vi "TLB Native Dynamic Events ver 0.09a.vi"() -> ()   [LabVIEW 2018]
uses:
  Labview Training Phase 2/Enum Controls/States for Action Engine.ctl
  Type def/TLB event states.ctl
  Type def/TLB MHL States.ctl
  <vilib>/Studica/Studica Toolkit/Background/I2C Channel.ctl
  <vilib>/myRIO/Common/Instrument Driver Framework/myRIO v1.0/AI/typedefs/AI Channels Enum.ctl
  <vilib>/myRIO/Common/Instrument Driver Framework/myRIO v1.0/AI/typedefs/AI Channels List.ctl
  Type def/Type def.ctl
  Underlying VI's/Webcam FGV Low level ver/State control.ctl
  <vilib>/userdefined/High Color/IMAQdx.ctl
  <vilib>/Studica/Studica Toolkit/NavX/NavX.lvlib
  <vilib>/Studica/Studica Toolkit/Background/DIO Channel.ctl
panel:
  out "State Queue Items":T1[](array[typedef])
  in  "NavX LED":bool
  out "Speed & distance":T2
  out "Motor Error":errorcluster
  in  "Direction":T3(ring)
  in  "Speed":dbl(slide) scale=-120.0..120.0
  out "I2C Error":errorcluster
  out "NavX Error":errorcluster
  out "Raw Values":T4
  out "NavX Data":T5
  out "Arduino Data":T6
  in  "STOP TASK":bool
  in  "Select task":i8
  in  "OK Button":bool
  out "Yaw":dbl
  out "Decision":i8
  in  "STOP":bool
  out "error out":errorcluster
  out "Object detection count":T7
  out "Camera error":errorcluster
  out "element":T1
  out "Action Queue Items":i32
  out "State Logic Queue Items":i32
  out "Action Queues items":string[](array[string])=["Hardware reset", "Software reset", ""]
  out "State logic":T8=enum."Task 2"
  out "Action State":string
  # "TLB FRAMEWORK STATUS"
  # "Camera Status Loop"
  # "Test Programme written by Calvin Loke    Dated: 28 Aug 2019\nTest Programme revised by Dr Alex See   Dated 30 Aug 2019\n\nProgramme version:   TLB Native Dynamic Events ver 0.04b.vi"
  # "Motor Control Loop"
  # "NAVX Control Loop"
  # "System Health Status Update"
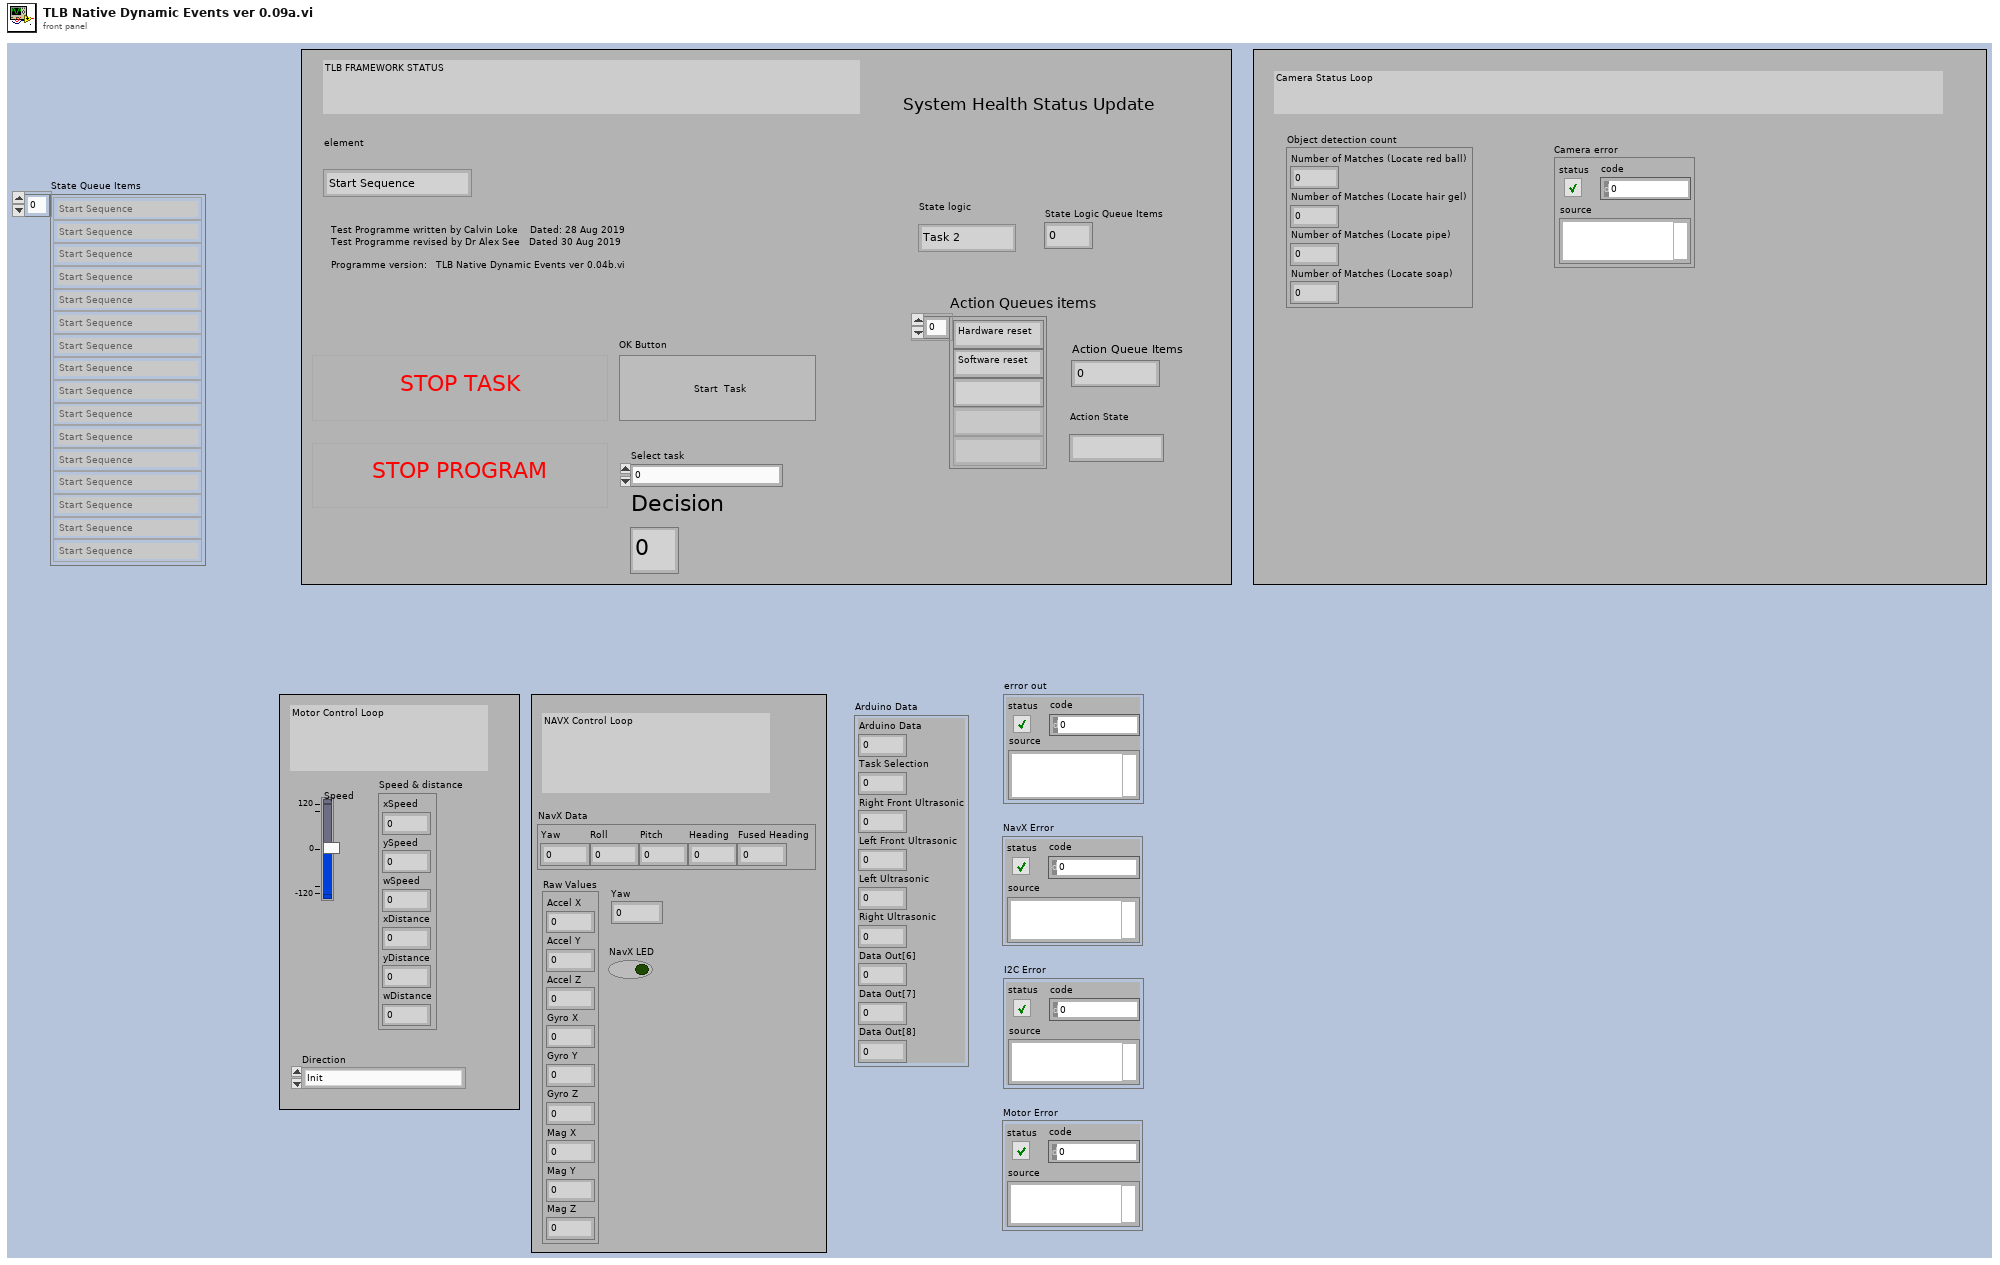
[diagram p1: front panel]
types:
  T1 = typedef "TLB event states.ctl" = enum16{"Start Sequence", "Exit", "Start Task 1", "Start Task 2", "Start Task 3", "Start Task 4", "Camera vision", "Wall follow mode", "Idle", "Start Drive Straight"}
  T2 = cluster{"xSpeed":dbl, "ySpeed":dbl, "wSpeed":dbl, "xDistance":dbl, "yDistance":dbl, "wDistance":dbl}
  T3 = enum16{"Init", "Front Back", "Left Right", "Rotate", "Latch"}
  T4 = cluster{"Accel X":dbl, "Accel Y":dbl, "Accel Z":dbl, "Gyro X":dbl, "Gyro Y":dbl, "Gyro Z":dbl, "Mag X":dbl, "Mag Y":dbl, "Mag Z":dbl}
  T5 = cluster{"Yaw":dbl, "Roll":dbl, "Pitch":dbl, "Heading":dbl, "Fused Heading":dbl}
  T6 = cluster{"Arduino Data":u8, "Task Selection":u8, "Right Front Ultrasonic":u8, "Left Front Ultrasonic":u8, "Left Ultrasonic":u8, "Right Ultrasonic":u8, "Data Out[6]":u8, "Data Out[7]":u8, "Data Out[8]":u8}
  T7 = cluster{"Number of Matches (Locate red ball)":i32, "Number of Matches (Locate hair gel)":i32, "Number of Matches (Locate pipe)":i32, "Number of Matches (Locate soap)":i32}
  T8 = typedef "TLB MHL States.ctl" = enum16{"None", "Startup", "Idle", "Processing", "Shutdown", "Reset", "Task 1", "Task 2", "Task 3", "Task 4", "Task 4a", "Task 4b", "Task 4c", "Task 4d", "Task 4e", "Task 4f", "Task 4g", "Task 4h", "Acquire image", "Wall follow mode", "Autodrive", "Autodrive a"}
  T9 = typedef "States for Action Engine.ctl" = enum16{"Initialize", "Write", "Read"}
  T10 = typedef "DIO Channel.ctl" = enum16{"Not Connected", "A/DIO1", "A/DIO2", "A/DIO3", "A/DIO4", "A/DIO5", "A/DIO6", "A/DIO7", "A/DIO13", "B/DIO1", "B/DIO2", "B/DIO3", "B/DIO4", "B/DIO5", "B/DIO6", "B/DIO7", "B/DIO13", "C/DIO0", "C/DIO1", "C/DIO2", "C/DIO3", "C/DIO4", "C/DIO5", "C/DIO6", "C/DIO7"}
  T11 = typedef "Type def.ctl" = cluster{"Front Ultrasonic Obstruct":bool, "Left Ultrasonic Obstruct":bool, "Right Ultrasonic Obstruct ":bool}
  T12 = typedef "I2C Channel.ctl" = enum16{"Not Connected", "A", "B"}
  T13 = typedef "State control.ctl" = enum16{"Initialise", "Start camera", "Continuous Acquisition ", "Stop camera", "Dispose all"}
  T14 = typedef "IMAQdx.ctl" = refnum<k21>
  T15 = cluster{"DIO Channel":T10, "FPGA VI Reference Out":refnum<k20>}
  T16 = typedef "AI Channels List.ctl" = T17[]
  T17 = typedef "AI Channels Enum.ctl" = enum16{"Not Connected", "AudioIn/Left", "AudioIn/Right", "C/AI0", "C/AI1", "A/AI0", "A/AI1", "A/AI2", "A/AI3", "A/AI4", "A/AI5", "A/AI6", "A/AI7", "B/AI0", "B/AI1", "B/AI2", "B/AI3", "B/AI4", "B/AI5", "B/AI6", "B/AI7", "AI/AI0", "AI/AI1", "AI/AI2", "AI/AI3", "A/AI0 (DIFF)", "A/AI1 (DIFF)", "A/AI2 (DIFF)", "A/AI3 (DIFF)", "B/AI0 (DIFF)", "B/AI1 (DIFF)", "B/AI2 (DIFF)", "B/AI3 (DIFF)"}
  T18 = cluster{"Arduino Status":u8, "Task Selection":u8, "PING_A":u8, "PING_B":u8, "PING_C":u8, "PING_D":u8, "Compass Low Byte":u8, "Compass High Byte":u8, "Data Out[8]":u8}
  T19 = cluster{"I2C Ref Out":cluster{"I2C Channel":T12, "FPGA VI Reference Out":refnum<k20>}, "Connected":bool, "Slave Address (7-bit)":u8, "Registry":u8[]}
  T20 = typedef "IMAQ Image.ctl" = refnum<image>
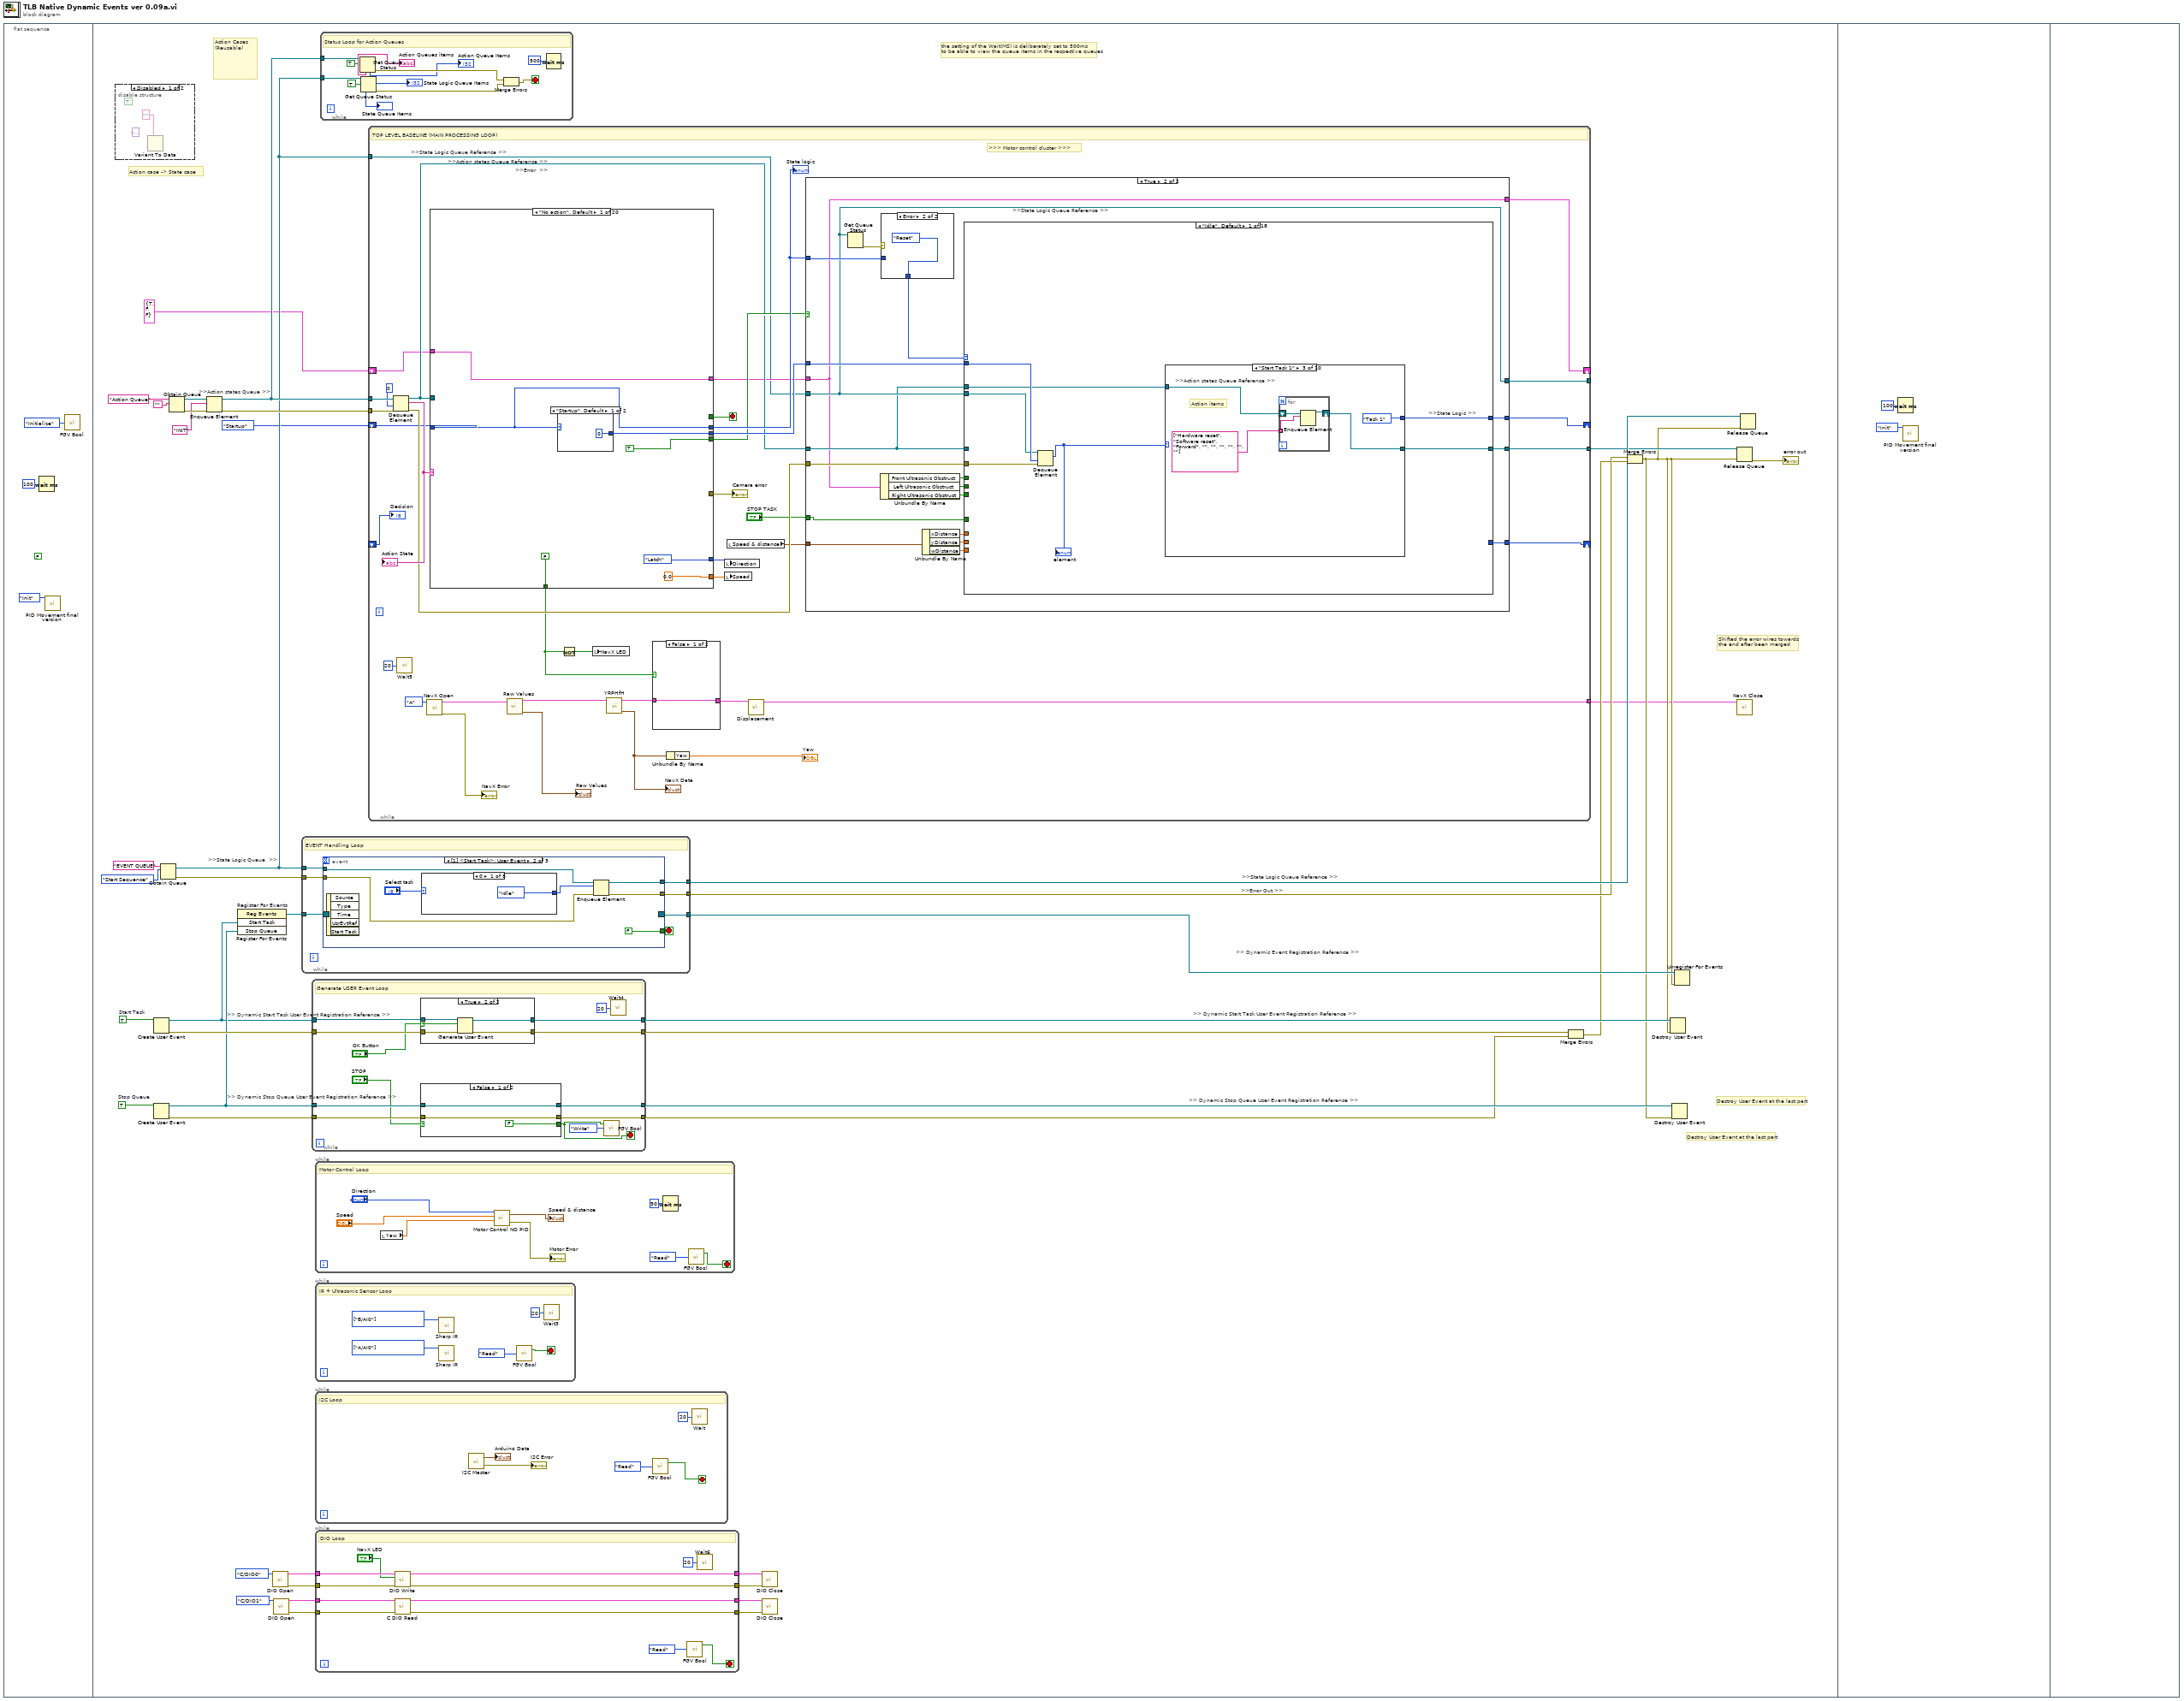
[diagram p0: block diagram]
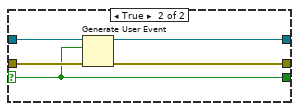
[diagram p3: hidden frame]
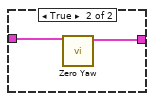
[diagram p5: hidden frame]
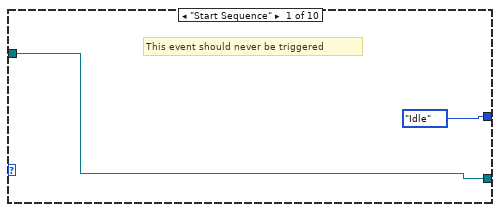
[diagram p8: hidden frame]
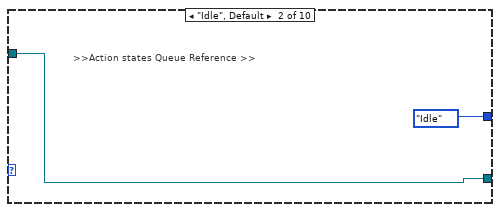
[diagram p9: hidden frame]
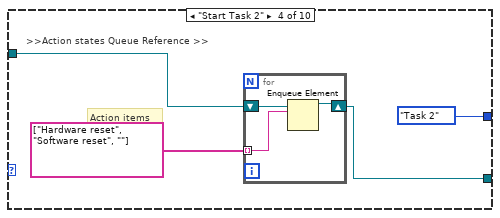
[diagram p10: hidden frame]
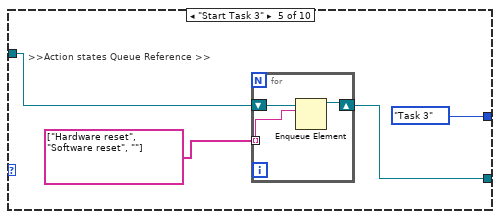
[diagram p11: hidden frame]
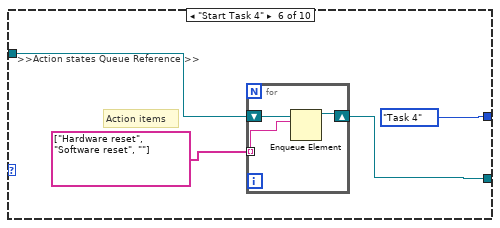
[diagram p12: hidden frame]
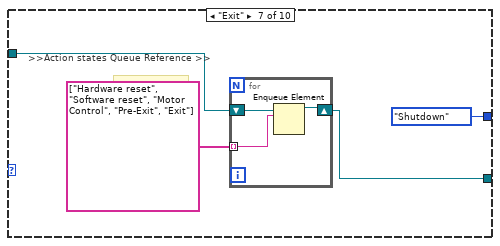
[diagram p13: hidden frame]
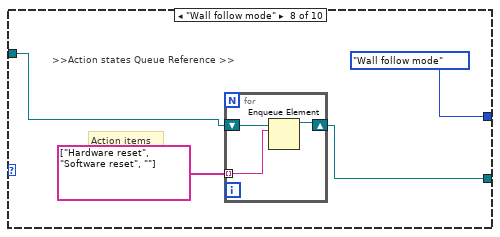
[diagram p14: hidden frame]
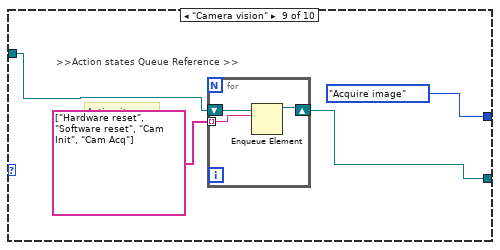
[diagram p15: hidden frame]
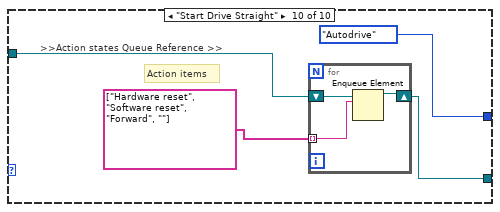
[diagram p16: hidden frame]
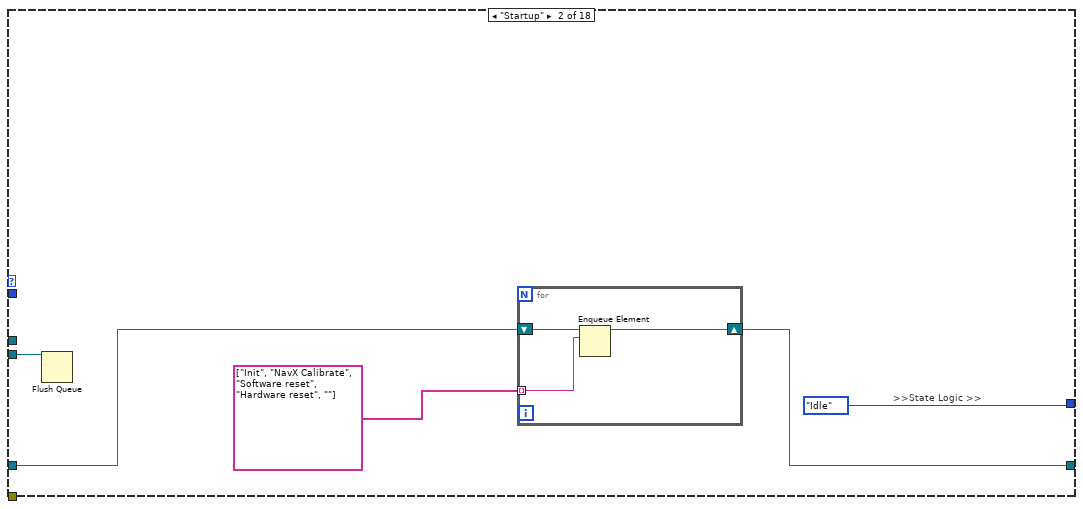
[diagram p17: hidden frame]
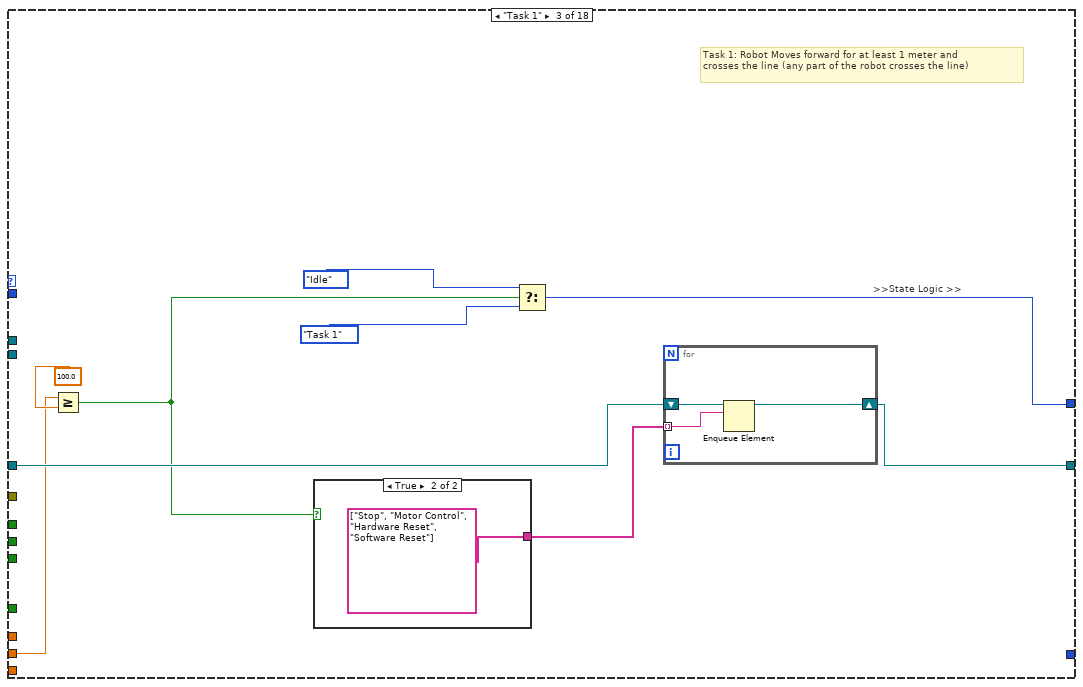
[diagram p18: hidden frame]
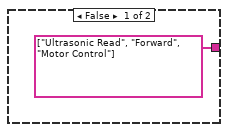
[diagram p19: hidden frame]
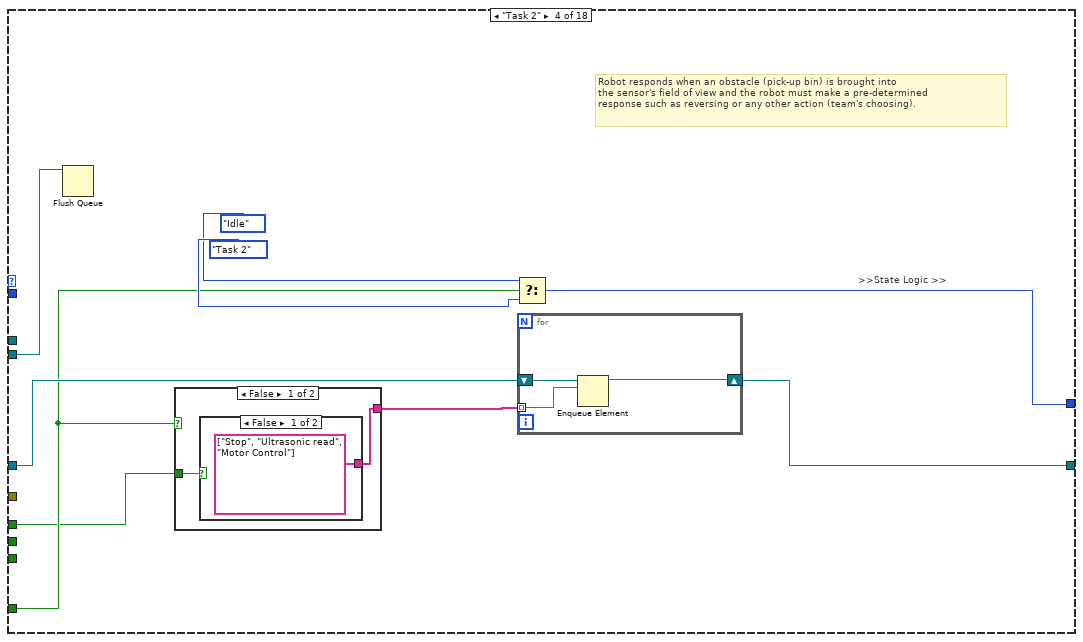
[diagram p20: hidden frame]
diagram:
  n1 = flat-sequence {
    frame #0 {
      (unwired) FALSE ("DIO 1")
      n2 = Wait (ms)(milliseconds to wait=u32 100) -> ()  [unwired: 1 out]
      n3 = call "PID Movement final version.vi"("Direction"=T3."Init") -> ()  [unwired: 3 in, 2 out]
      n4 = call "FGV Bool.vi"("Init/Read/Write State"=States_for_Action_Engine."Initialize") -> ()  [unwired: 2 in, 2 out]
    }
    frame #1 {
      w45 = TRUE  # Stop Queue
      w44 = TRUE  # Start Task
      # "Action case -> State case"
      # "the setting of the Wait(MS) is deliberately set to 500ms\nto be able to view the queue items in the respective queues"
      # "Action Cases\n(Reusable)"
      # ">>Error Out >>"
      # ">> Dynamic Stop Queue User Event Registration Reference >>"
      # ">> Dynamic Start Task User Event Registration Reference >>"
      # ">> Dynamic Stop Queue User Event Registration Reference >>"
      # ">> Dynamic Start Task User Event Registration Reference >>"
      # ">> Dynamic Event Registration Reference >>"
      # ">>Action states Queue >>"
      # ">>State Logic Queue  >>"
      # ">>State Logic Queue Reference >>"
      # "Destroy User Event at the last part"
      # "Destroy User Event at the last part"
      # "Shifted the error wires towards\nthe end after been merged"
      n5 = disable-structure shown="Disabled" {
        frame Disabled {
          (unwired) variant
          (unwired) TRUE
          n6 = Variant To Data(type="") -> ()  [unwired: 2 in, 2 out]
        }
        frame Enabled {
        }
      }
      n7 = Create User Event(user event datatype=w44) -> (user event=w36:refnum<user-event>, error out=w41:errorcluster)  [unwired: 1 in]
      n8 = Create User Event(user event datatype=w45) -> (user event=w37:refnum<user-event>, error out=w40:errorcluster)  [unwired: 1 in]
      n9 = Obtain Queue(name (unnamed)="EVENT QUEUE", element data type=TLB_event_states."Start Sequence" ("Enum")) -> (queue out=w21:refnum<queue>, error out=w27:errorcluster)  [unwired: 3 in, 1 out]
      n10 = Obtain Queue(name (unnamed)="Action Queue", element data type="") -> (queue out=w30:refnum<queue>, error out=w26:errorcluster)  [unwired: 3 in, 1 out]
      n11 = Enqueue Element(queue=w30, element="INIT", error in (no error)=w26) -> (queue out=w22:refnum<queue>, error out=w25:errorcluster)  [unwired: 1 in, 1 out]
      n12 = register-events "Register For Events"(w36, w37) -> (reference out=w35:refnum<event-registration>)  [unwired: 2 in, 1 out]
      n13 = call <vilib>:"DIO Open.vi"("DIO Channel"=DIO_Channel."C/DIO0") -> ("error out"=w11:errorcluster, "DIO Info Out"=w13:T15)  [unwired: 9 in]
      n14 = call <vilib>:"DIO Open.vi"("DIO Channel"=DIO_Channel."C/DIO1") -> ("error out"=w7:errorcluster, "DIO Info Out"=w8:T15)  [unwired: 9 in]
      n15 = while {
        tunnel: w35 -> [w637]
        tunnel: [w636] -> w34
        tunnel: w21 -> [w634]
        tunnel: [w633] -> w33
        tunnel: w27 -> [w632]
        tunnel: [w631] -> w24
        stop <- w635 stop-if-true
        # "EVENT Handling Loop"
        n16 = event shown="[1] <Start Task>: User Event" {
          selector: w637 -> [_ _ _]
          dyn-events: [_ _ _] -> w636
          timeout: _ -> [_ _ _]
          tunnel: [FALSE FALSE w664] -> w635
          tunnel: w634 -> [w642 w649 w662]
          tunnel: [w641 w648 w663] -> w633
          tunnel: w632 -> [w639 w647 w660]
          tunnel: [w638 w646 w659] -> w631
          event Timeout {
            n17 = event-data() -> ()  [unwired: 1 in, 3 out]
            n18 = Enqueue Element(queue=w642, element=TLB_event_states."Idle" ("Enum"), error in (no error)=w639) -> (queue out=w641:refnum<queue>, error out=w638:errorcluster)  [unwired: 1 in, 1 out]
          }
          event User Event {
            n19 = event-data() -> ()  [unwired: 1 in, 5 out]
            n20 = case shown="0" "Select task" {
              tunnel: [TLB_event_states."Idle" ("Enum") TLB_event_states."Start Task 1" ("Enum") TLB_event_states."Start Task 2" ("Enum") TLB_event_states."Start Task 3" ("Enum") TLB_event_states."Start Task 4" ("Enum") TLB_event_states."Wall follow mode" ("Enum") TLB_event_states."Camera vision" ("Enum") TLB_event_states."Start Drive Straight" ("Enum")] -> w645
              frame 0 {
              }
              frame 1 {
              }
              frame 2 {
              }
              frame 3, Default {
              }
              frame 4 {
              }
              frame 5 {
              }
              frame 6 {
              }
              frame 7 {
              }
            }
            n21 = Enqueue Element(queue=w649, element=w645, error in (no error)=w647) -> (queue out=w648:refnum<queue>, error out=w646:errorcluster)  [unwired: 1 in, 1 out]
          }
          event User Event {
            n22 = event-data() -> ("Stop Queue"=w664:bool)  [unwired: 1 in, 4 out]
            n23 = Enqueue Element At Opposite End(queue=w662, element=TLB_event_states."Exit" ("Enum"), error in (no error)=w660) -> (queue out=w663:refnum<queue>, error out=w659:errorcluster)  [unwired: 1 in, 1 out]
          }
        }
      }
      n24 = while {
        tunnel: w36 -> [w96]
        tunnel: w37 -> [w95]
        tunnel: [w94] -> w43
        tunnel: [w93] -> w42
        tunnel: w41 -> [w92]
        tunnel: [w91] -> w39
        tunnel: w40 -> [w90]
        tunnel: [w89] -> w38
        stop <- w87 stop-if-true
        # "Generate USER Event Loop"
        n25 = case shown="True" "OK Button" {
          selector: "OK Button" -> [_ w107]
          tunnel: w96 -> [w106 w111]
          tunnel: [w106 w110] -> w93
          tunnel: w92 -> [w105 w109]
          tunnel: [w105 w108] -> w91
          frame False {
          }
          frame True {
            n26 = Generate User Event(user event=w111, event data cluster=w107, error in=w109) -> (user event out=w110:refnum<user-event>, error out=w108:errorcluster)  [unwired: 1 in]
          }
        }
        n27 = case shown="False" "STOP" {
          selector: "STOP" -> [_ w100]
          tunnel: w95 -> [w99 w104]
          tunnel: [w99 w103] -> w94
          tunnel: w90 -> [w98 w102]
          tunnel: [w98 w101] -> w89
          tunnel: [FALSE w100] -> w87
          frame False {
          }
          frame True {
            n28 = Generate User Event(user event=w104, event data cluster=w100, error in=w102) -> (user event out=w103:refnum<user-event>, error out=w101:errorcluster)  [unwired: 1 in]
          }
        }
        n29 = call "FGV Bool.vi"("Init/Read/Write State"=States_for_Action_Engine."Write", "Input Node"=w87) -> ()  [unwired: 1 in, 2 out]
        n30 = call "Wait4"("Count(uSec)"=u32 20) -> ()  [unwired: 1 out]
      }
      n31 = while {
        stop <- w64 stop-if-true
        # "Motor Control Loop"
        n32 = local read "Yaw"() -> (w60:dbl)
        n33 = call "Motor Control NO PID.vi"("Yaw"=w60, "Speed"="Speed", "Direction"="Direction") -> ("error out"=→"Motor Error":errorcluster, "Speed & distance"=→"Speed & distance":T2)  [unwired: 1 in]
        n34 = Wait (ms)(milliseconds to wait=u32 50) -> ()  [unwired: 1 out]
        n35 = call "FGV Bool.vi"("Init/Read/Write State"=States_for_Action_Engine."Read") -> ("Output node"=w64:bool)  [unwired: 2 in, 1 out]
      }
      n36 = while {
        stop <- w627 stop-if-true
        w629 = T16 [enum."A/AI0"] items=["Not Connected", "AudioIn/Left", "AudioIn/Right", "C/AI0", "C/AI1", "A/AI0", "A/AI1", "A/AI2", "A/AI3", "A/AI4", "A/AI5", "A/AI6", "A/AI7", "B/AI0", "B/AI1", "B/AI2", "B/AI3", "B/AI4", "B/AI5", "B/AI6", "B/AI7", "AI/AI0", "AI/AI1", "AI/AI2", "AI/AI3", "A/AI0 (DIFF)", "A/AI1 (DIFF)", "A/AI2 (DIFF)", "A/AI3 (DIFF)", "B/AI0 (DIFF)", "B/AI1 (DIFF)", "B/AI2 (DIFF)", "B/AI3 (DIFF)"] ("AI Channel")
        w630 = T16 [enum."B/AI0"] items=["Not Connected", "AudioIn/Left", "AudioIn/Right", "C/AI0", "C/AI1", "A/AI0", "A/AI1", "A/AI2", "A/AI3", "A/AI4", "A/AI5", "A/AI6", "A/AI7", "B/AI0", "B/AI1", "B/AI2", "B/AI3", "B/AI4", "B/AI5", "B/AI6", "B/AI7", "AI/AI0", "AI/AI1", "AI/AI2", "AI/AI3", "A/AI0 (DIFF)", "A/AI1 (DIFF)", "A/AI2 (DIFF)", "A/AI3 (DIFF)", "B/AI0 (DIFF)", "B/AI1 (DIFF)", "B/AI2 (DIFF)", "B/AI3 (DIFF)"] ("AI Channel")
        # "IR + Ultrasonic Sensor Loop"
        n37 = call <vilib>:"Sharp IR.vi"("AI Channel"=w630) -> ()  [unwired: 8 in, 3 out]
        n38 = call <vilib>:"Sharp IR.vi"("AI Channel"=w629) -> ()  [unwired: 8 in, 3 out]
        n39 = call "FGV Bool.vi"("Init/Read/Write State"=States_for_Action_Engine."Read") -> ("Output node"=w627:bool)  [unwired: 2 in, 1 out]
        n40 = call "Wait3"("Count(uSec)"=u32 20) -> ()  [unwired: 1 out]
      }
      n41 = while {
        stop <- w69 stop-if-true
        # "I2C Loop"
        n42 = call "I2C Master.vi"() -> ("I2C Error"=→"I2C Error":errorcluster, "Arduino Data"=→"Arduino Data":T18)  [unwired: 2 in]
        n43 = call "FGV Bool.vi"("Init/Read/Write State"=States_for_Action_Engine."Read") -> ("Output node"=w69:bool)  [unwired: 2 in, 1 out]
        n44 = call "Wait"("Count(uSec)"=u32 20) -> ()  [unwired: 1 out]
      }
      n45 = while {
        tunnel: w13 -> [w54]
        tunnel: [w53] -> w12
        tunnel: w11 -> [w52]
        tunnel: [w51] -> w10
        tunnel: [w50] -> w9
        tunnel: w8 -> [w49]
        tunnel: w7 -> [w48]
        tunnel: [w47] -> w6
        stop <- w56 stop-if-true
        # "DIO Loop"
        n46 = call <vilib>:"DIO Write.vi"("error in (no error)"=w52, "Input"="NavX LED", "DIO Info In"=w54) -> ("error out"=w51:errorcluster, "DIO Info Out"=w53:T15)  [unwired: 7 in]
        n47 = call <vilib>:"C DIO Read.vi"("error in (no error)"=w48, "DIO Info In in"=w49) -> ("error out"=w47:errorcluster, "DIO Info In out"=w50:T15)  [unwired: 7 in, 1 out]
        n48 = call "FGV Bool.vi"("Init/Read/Write State"=States_for_Action_Engine."Read") -> ("Output node"=w56:bool)  [unwired: 2 in, 1 out]
        n49 = call "Wait6"("Count(uSec)"=u32 20) -> ()  [unwired: 1 out]
      }
      n50 = while {
        tunnel: w22 -> [w81]
        tunnel: w21 -> [w78]
        stop <- w75 stop-if-true
        # "Status Loop for Action Queues"
        n51 = Get Queue Status(queue=w81, return elements? (F)=TRUE) -> (error out=w77:errorcluster, # elements in queue=→"Action Queue Items":i32, elements=→"Action Queues items":string[])  [unwired: 1 in, 5 out]
        n52 = Get Queue Status(queue=w78, return elements? (F)=TRUE) -> (# pending remove=→"State Logic Queue Items":i32, error out=w76:errorcluster, elements=→"State Queue Items":T1[])  [unwired: 1 in, 5 out]
        n53 = Merge Errors(w77, w76) -> (w75:errorcluster)
        n54 = Wait (ms)(milliseconds to wait=u32 500) -> ()  [unwired: 1 out]
      }
      n55 = while {
        tunnel: w21 -> [w132]
        shift-right: [w143] -> _
        shift-left: TLB_MHL_States."Startup" ("Enum") -> [w137]
        tunnel: w22 -> [w148]
        tunnel: w25 -> [w146]
        tunnel: [w145] -> _
        tunnel: [w144] -> w17
        shift-right: [w134] -> _
        shift-left: T11 {"Front Ultrasonic Obstruct"=TRUE, "Left Ultrasonic Obstruct"=FALSE, "Right Ultrasonic Obstruct "=FALSE} -> [w136]
        shift-right: [w130] -> _
        shift-left: _ -> [w129]
        tunnel: [w122] -> w14
        stop <- w131 stop-if-true
        # ">>> Motor control cluster >>>"
        # ">>Error  >>"
        # ">>Action states Queue Reference >>"
        # ">>State Logic Queue Reference >>"
        # "TOP LEVEL BASELINE (MAIN PROCESSING LOOP)"
        n56 = Dequeue Element(queue=w148, timeout in ms (-1)=0, error in (no error)=w146) -> (queue out=w138:refnum<queue>, element=w147:string, error out=w139:errorcluster)  [unwired: 1 out]
        "Action State" <- w147
        n57 = call "Wait5"("Count(uSec)"=u32 20) -> ()  [unwired: 1 out]
        n58 = call <vilib>:"NavX Open.vi"("I2C Channel"=I2C_Channel."A") -> ("error out"=→"NavX Error":errorcluster, "NavX Info"=w124:T19)  [unwired: 9 in]
        n59 = case shown="\"No action\", Default" w147 {
          tunnel: [w463 w476 w481 w487 w494 w500 w504 w512 w518 w524 w535 w543 TLB_MHL_States."Shutdown" ("Enum") w555 w578 w584 w595 w605 w618 w624] -> w149
          tunnel: [w466 0 0 0 0 0 0 0 0 0 0 0 0 0 0 0 0 0 0 0] -> w142
          tunnel: [TRUE FALSE FALSE FALSE FALSE FALSE FALSE FALSE FALSE FALSE FALSE FALSE FALSE FALSE FALSE FALSE FALSE FALSE FALSE FALSE] -> w141
          tunnel: w138 -> [_ _ _ _ _ _ _ _ _ _ _ _ _ _ _ _ _ _ _ _]
          tunnel: w137 -> [w463 w476 w481 w487 w494 w500 w504 w512 w518 w524 w535 w543 _ w555 w578 w584 w595 w605 w618 w624]
          tunnel: w136 -> [w464 w472 w479 w485 w491 w497 w503 w509 w516 w525 w530 w540 w547 w556 w574 w581 w596 w604 w615 w625]
          tunnel: [w464 w473 w479 w485 w491 w497 w503 w509 w516 w525 w529 w540 w547 w556 w575 w581 w596 w604 w615 w625] -> w135
          tunnel: [_ _ _ _ _ _ _ _ _ _ _ _ _ _ _ _ w587 w600 w610 _] -> w133
          tunnel: [_ _ _ _ _ _ _ _ _ _ _ _ TRUE _ _ _ _ _ _ _] -> w131
          tunnel: [FALSE ("NavX Zero Yaw") _ _ _ _ _ _ _ FALSE ("NavX Zero Yaw") _ FALSE ("NavX Zero Yaw") TRUE ("NavX Zero Yaw") _ _ _ _ _ _ _ _] -> w112
          tunnel: [T3."Latch" ("Direction") T3."Init" ("Direction") T3."Front Back" ("Direction") T3."Front Back" ("Direction") T3."Left Right" ("Direction") T3."Left Right" ("Direction") T3."Rotate" ("Direction") T3."Rotate" ("Direction") T3."Front Back" ("Direction") T3."Latch" ("Direction") T3."Init" ("Direction") T3."Init" ("Direction") T3."Init" ("Direction") T3."Init" ("Direction") T3."Latch" ("Direction") T3."Latch" ("Direction") T3."Latch" ("Direction") T3."Latch" ("Direction") T3."Latch" ("Direction") T3."Init" ("Direction")] -> w116
          tunnel: [0.0 0.0 0.8 -50.0 50.0 -50.0 50.0 -50.0 0.0 0.0 0.0 0.0 0.0 0.0 0.0 0.0 0.0 0.0 0.0 0.0] -> w115
          frame "No action", Default {
            n60 = case shown="\"Startup\", Default" w463 {
              tunnel: [0 100] -> w466
              frame "Startup", Default {
              }
              frame "Idle" {
              }
            }
          }
          frame "Init" {
            w471 = FALSE ("Object detected")
            # ">>State Logic  >>"
            n61 = Bundle By Name(cluster=w472, "Front Ultrasonic Obstruct"=w471, "Left Ultrasonic Obstruct"=w471, "Right Ultrasonic Obstruct"=w471) -> (w473:T11)
          }
          frame "Forward" {
          }
          frame "Reverse" {
          }
          frame "Right" {
          }
          frame "Left" {
          }
          frame "Rotate CW" {
          }
          frame "Rotate ACW" {
          }
          frame "Stop" {
          }
          frame "Motor Control" {
          }
          frame "Software reset" {
            w528 = FALSE
            # "Resets any software variables\nand/or non-critical states"
            n62 = Wait (ms)(milliseconds to wait=u32 20) -> ()  [unwired: 1 out]
            n63 = Bundle By Name(cluster=w530, "Front Ultrasonic Obstruct"=w528, "Left Ultrasonic Obstruct"=w528, "Right Ultrasonic Obstruct"=w528) -> (w529:T11)
          }
          frame "Hardware reset" {
            n64 = Wait (ms)(milliseconds to wait=u32 100) -> ()  [unwired: 1 out]
          }
          frame "Exit" {
          }
          frame "Pre-Exit" {
          }
          frame "Ultrasonic read" {
            w565 = 10.0 ("y")
            # "Object detection"
            n65 = local read "Arduino Data"() -> (w573:T6)
            n66 = Unbundle By Name(w573) -> ("Right Front Ultrasonic"=w560:u8, "Left Front Ultrasonic"=w559:u8, "Left Ultrasonic"=w567:u8, "Right Ultrasonic"=w566:u8)
            n67 = To Double Precision Float(number=w559) -> (double precision float=w558:dbl)
            n68 = To Double Precision Float(number=w560) -> (double precision float=w557:dbl)
            n69 = Less?(x=w567, y=w565) -> (x < y?=w564:bool)
            n70 = Less?(x=w566, y=w565) -> (x < y?=w563:bool)
            n71 = Add(x=w557, y=w558) -> (x+y=w572:dbl)
            n72 = Divide(x=w572, y=u8 2) -> (x/y=w570:dbl)
            n73 = Less?(x=w570, y=20.0) -> (x < y?=w568:bool)
            n74 = Bundle By Name(cluster=w574, "Front Ultrasonic Obstruct"=w568, "Left Ultrasonic Obstruct"=w564, "Right Ultrasonic Obstruct"=w563) -> (w575:T11)
          }
          frame "IR Sensor Read" {
          }
          frame "Cam Init" {
            n75 = call "Low-Level Grab.vi"("States"=State_control."Initialise", "Session In"=T14 "cam1") -> ("error out"=w588:errorcluster, "Session Out"=w589:T14)  [unwired: 7 in, 1 out]
            n76 = call "Low-Level Grab.vi"("error in (no error)"=w588, "States"=State_control."Start camera", "Session In"=w589) -> ("error out"=w587:errorcluster)  [unwired: 6 in, 2 out]
          }
          frame "Cam Acq" {
            n77 = call "Low-Level Grab.vi"("States"=State_control."Continuous Acquisition ") -> ("error out"=w601:errorcluster, "Image Out"=w602:T20)  [unwired: 8 in, 1 out]
            n78 = call "All object detection ver2.vi"("Image In"=w602, "error in"=w601) -> ("Object detection count"=→"Object detection count":T7, "error out"=w600:errorcluster)  [unwired: 1 out]
          }
          frame "Cam Exit" {
            n79 = call "Low-Level Grab.vi"("States"=State_control."Stop camera") -> ("error out"=w611:errorcluster, "Session Out"=w613:T14)  [unwired: 8 in, 1 out]
            n80 = call "Low-Level Grab.vi"("error in (no error)"=w611, "States"=State_control."Dispose all", "Session In"=w613) -> ("error out"=w610:errorcluster)  [unwired: 6 in, 2 out]
          }
          frame "NavX Calibrate" {
            # "Adds a 15 second delay to the startup process \nfor the NavX to calibrate"
            n81 = Wait (ms)(milliseconds to wait=u32 15000) -> ()  [unwired: 1 out]
          }
        }
        "State logic" <- w149
        "Camera error" <- w133
        n82 = call <vilib>:"Raw Values.vi"("NavX Info In"=w124) -> ("Raw Values"=→"Raw Values":T4, "NavX Info Out"=w127:T19)  [unwired: 8 in]
        n83 = Not(x=w112) -> (.not. x?=w113:bool)
        n84 = local write "NavX LED"(w113) -> ()
        n85 = call <vilib>:"YRPHfH.vi"("NavX Info In"=w127) -> ("YRPHfH"=w128:T5, "NavX Info Out"=w126:T19)  [unwired: 3 in]
        "NavX Data" <- w128
        n86 = case shown="False" w112 {
          tunnel: [w150 w152] -> w123
          tunnel: w126 -> [w150 w151]
          frame False {
          }
          frame True {
            n87 = call <vilib>:"Zero Yaw.vi"("NavX Info In"=w151) -> ("NavX Info Out"=w152:T19)  [unwired: 10 in]
          }
        }
        n88 = Unbundle By Name(w128) -> ("Yaw"=→"Yaw":dbl)
        n89 = local write "Direction"(w116) -> ()
        n90 = local write "Speed"(w115) -> ()
        n91 = local read "Speed & distance"() -> (w117:T2)
        n92 = call <vilib>:"Displacement.vi"("NavX Info In"=w123) -> ("NavX Info Out"=w122:T19)  [unwired: 9 in, 1 out]
        n93 = case shown="True" w141 {
          tunnel: w149 -> [w155 w170]
          tunnel: w132 -> [w156 w169]
          tunnel: w138 -> [w154 w167]
          tunnel: [w156 w169] -> w145
          tunnel: [w154 w175] -> w144
          tunnel: [w155 w174] -> w143
          tunnel: w139 -> [_ w173]
          tunnel: w142 -> [_ w172]
          tunnel: w135 -> [w153 w161]
          tunnel: [w153 w161] -> w134
          tunnel: [_ w166] -> w130
          tunnel: "STOP TASK" -> [_ w165]
          tunnel: w117 -> [_ w157]
          frame False {
          }
          frame True {
            # ">>State Logic Queue Reference >>"
            n94 = Get Queue Status(queue=w169) -> (error out=w168:errorcluster)  [unwired: 2 in, 7 out]
            n95 = Unbundle By Name(w161) -> ("Front Ultrasonic Obstruct"=w160:bool, "Left Ultrasonic Obstruct"=w159:bool, "Right Ultrasonic Obstruct"=w158:bool)
            n96 = case shown="Error" w168 {
              tunnel: [w176 TLB_MHL_States."Reset" ("Enum")] -> w171
              tunnel: w170 -> [w176 _]
              frame No Error {
              }
              frame Error {
              }
            }
            n97 = Unbundle By Name(w157) -> ("xDistance"=w162:dbl, "yDistance"=w164:dbl, "wDistance"=w163:dbl)
            n98 = case shown="\"Idle\", Default" w171 {
              tunnel: w169 -> [w180 w246 _ w269 w287 w304 w319 w334 w349 w365 _ w386 w405 _ w437 _ _ _]
              tunnel: w167 -> [_ w248 w257 w271 w294 w306 w323 w339 w353 w369 w379 w388 w406 w429 w440 w449 w452 w458]
              tunnel: [w178 w247 w256 w272 w293 w307 w322 w338 w352 w368 w378 w389 w407 w430 w439 w449 w451 w458] -> w175
              tunnel: [w183 TLB_MHL_States."Idle" ("Enum") w259 w273 w290 w310 w325 w337 w354 w367 TLB_MHL_States."Shutdown" ("Enum") w391 w401 w426 w438 TLB_MHL_States."Reset" ("Enum") TLB_MHL_States."Shutdown" ("Enum") TLB_MHL_States."Reset" ("Enum")] -> w174
              tunnel: w173 -> [w181 _ _ _ _ _ _ _ _ _ _ _ _ _ _ _ _ _]
              tunnel: w172 -> [w182 _ _ _ _ _ _ _ _ _ _ _ _ _ _ _ _ _]
              tunnel: w167 -> [w179 _ _ _ _ _ _ _ _ _ _ _ _ _ _ _ _ _]
              tunnel: [_ _ _ _ _ _ _ _ _ _ _ _ w400 _ _ _ _ _] -> w166
              tunnel: w165 -> [_ _ _ w268 w285 w301 _ _ _ w364 _ w385 w399 w418 w436 _ _ _]
              tunnel: w164 -> [_ _ w253 _ _ _ w318 _ _ _ _ _ _ w417 _ _ _ _]
              tunnel: w163 -> [_ _ _ _ w284 _ _ _ _ _ _ _ _ _ _ _ _ _]
              tunnel: w162 -> [_ _ _ _ _ _ _ w333 w348 _ _ _ _ _ _ _ _ _]
              tunnel: w160 -> [_ _ _ w267 _ w302 _ _ _ w363 _ _ w398 _ _ _ _ _]
              tunnel: w159 -> [_ _ _ _ _ _ _ _ _ _ _ _ _ _ _ _ _ _]
              tunnel: w158 -> [_ _ _ _ _ _ _ _ _ _ _ _ _ _ _ _ _ _]
              frame "Idle", Default {
                # ">>State Logic >>"
                n99 = Dequeue Element(queue=w180, timeout in ms (-1)=w182, error in (no error)=w181) -> (element=w184:T1)  [unwired: 3 out]
                "element" <- w184
                n100 = case shown="\"Start Task 1\"" w184 {
                  tunnel: [TLB_MHL_States."Idle" ("Enum") TLB_MHL_States."Idle" ("Enum") TLB_MHL_States."Task 1" ("Enum") TLB_MHL_States."Task 2" ("Enum") TLB_MHL_States."Task 3" ("Enum") TLB_MHL_States."Task 4" ("Enum") TLB_MHL_States."Shutdown" ("Enum") TLB_MHL_States."Wall follow mode" ("Enum") TLB_MHL_States."Acquire image" ("Enum") TLB_MHL_States."Autodrive" ("Enum")] -> w183
                  tunnel: w179 -> [w185 w187 w191 w198 w204 w212 w219 w226 w233 w240]
                  tunnel: [w185 w187 w190 w197 w205 w211 w218 w225 w232 w238] -> w178
                  frame "Start Sequence" {
                    # "This event should never be triggered"
                  }
                  frame "Idle", Default {
                    # ">>Action states Queue Reference >>"
                  }
                  frame "Start Task 1" {
                    # ">>Action states Queue Reference >>"
                    # "Action items"
                    n101 = for {
                      shift-right: [w195] -> w190
                      shift-left: w191 -> [w194]
                      tunnel: string[] ["Hardware reset", "Software reset", "Forward", "", "", "", "", "", ""] -> [w193] mode=indexing
                      n102 = Enqueue Element(queue=w194, element=w193) -> (queue out=w195:refnum<queue>)  [unwired: 2 in, 2 out]
                    }
                  }
                  frame "Start Task 2" {
                    # ">>Action states Queue Reference >>"
                    # "Action items"
                    n103 = for {
                      shift-right: [w202] -> w197
                      shift-left: w198 -> [w201]
                      tunnel: string[] ["Hardware reset", "Software reset", ""] -> [w200] mode=indexing
                      n104 = Enqueue Element(queue=w201, element=w200) -> (queue out=w202:refnum<queue>)  [unwired: 2 in, 2 out]
                    }
                  }
                  frame "Start Task 3" {
                    # ">>Action states Queue Reference >>"
                    n105 = for {
                      shift-right: [w209] -> w205
                      shift-left: w204 -> [w208]
                      tunnel: string[] ["Hardware reset", "Software reset", ""] -> [w207] mode=indexing
                      n106 = Enqueue Element(queue=w208, element=w207) -> (queue out=w209:refnum<queue>)  [unwired: 2 in, 2 out]
                    }
                  }
                  frame "Start Task 4" {
                    # ">>Action states Queue Reference >>"
                    # "Action items"
                    n107 = for {
                      shift-right: [w216] -> w211
                      shift-left: w212 -> [w215]
                      tunnel: string[] ["Hardware reset", "Software reset", ""] -> [w214] mode=indexing
                      n108 = Enqueue Element(queue=w215, element=w214) -> (queue out=w216:refnum<queue>)  [unwired: 2 in, 2 out]
                    }
                  }
                  frame "Exit" {
                    # ">>Action states Queue Reference >>"
                    # "Action items"
                    n109 = for {
                      shift-right: [w223] -> w218
                      shift-left: w219 -> [w222]
                      tunnel: string[] ["Hardware reset", "Software reset", "Motor Control", "Pre-Exit", "Exit"] -> [w221] mode=indexing
                      n110 = Enqueue Element(queue=w222, element=w221) -> (queue out=w223:refnum<queue>)  [unwired: 2 in, 2 out]
                    }
                  }
                  frame "Wall follow mode" {
                    # ">>Action states Queue Reference >>"
                    # "Action items"
                    n111 = for {
                      shift-right: [w230] -> w225
                      shift-left: w226 -> [w229]
                      tunnel: string[] ["Hardware reset", "Software reset", ""] -> [w228] mode=indexing
                      n112 = Enqueue Element(queue=w229, element=w228) -> (queue out=w230:refnum<queue>)  [unwired: 2 in, 2 out]
                    }
                  }
                  frame "Camera vision" {
                    # ">>Action states Queue Reference >>"
                    # "Action items"
                    n113 = for {
                      shift-right: [w237] -> w232
                      shift-left: w233 -> [w236]
                      tunnel: string[] ["Hardware reset", "Software reset", "Cam Init", "Cam Acq"] -> [w235] mode=indexing
                      n114 = Enqueue Element(queue=w236, element=w235) -> (queue out=w237:refnum<queue>)  [unwired: 2 in, 2 out]
                    }
                  }
                  frame "Start Drive Straight" {
                    # ">>Action states Queue Reference >>"
                    # "Action items"
                    n115 = for {
                      shift-right: [w244] -> w238
                      shift-left: w240 -> [w243]
                      tunnel: string[] ["Hardware reset", "Software reset", "Forward", ""] -> [w242] mode=indexing
                      n116 = Enqueue Element(queue=w243, element=w242) -> (queue out=w244:refnum<queue>)  [unwired: 2 in, 2 out]
                    }
                  }
                }
              }
              frame "Startup" {
                # ">>State Logic >>"
                n117 = Flush Queue(queue=w246) -> ()  [unwired: 1 in, 3 out]
                n118 = for {
                  shift-right: [w251] -> w247
                  shift-left: w248 -> [w252]
                  tunnel: string[] ["Init", "NavX Calibrate", "Software reset", "Hardware reset", ""] -> [w250] mode=indexing
                  n119 = Enqueue Element(queue=w252, element=w250) -> (queue out=w251:refnum<queue>)  [unwired: 2 in, 2 out]
                }
              }
              frame "Task 1" {
                # "Task 1: Robot Moves forward for at least 1 meter and\ncrosses the line (any part of the robot crosses the line)"
                # ">>State Logic >>"
                n120 = Greater Or Equal?(x=w253, y=100.0) -> (x >= y?=w254:bool)
                n121 = case shown="True" w254 {
                  tunnel: [string[] ["Ultrasonic Read", "Forward", "Motor Control"] string[] ["Stop", "Motor Control", "Hardware Reset", "Software Reset"]] -> w258
                  frame False {
                  }
                  frame True {
                  }
                }
                n122 = Select(t=TLB_MHL_States."Idle" ("Enum"), s=w254, f=TLB_MHL_States."Task 1" ("Enum")) -> (s? t:f=w259:T8)
                n123 = for {
                  shift-right: [w265] -> w256
                  shift-left: w257 -> [w266]
                  tunnel: w258 -> [w264] mode=indexing
                  n124 = Enqueue Element(queue=w266, element=w264) -> (queue out=w265:refnum<queue>)  [unwired: 2 in, 2 out]
                }
              }
              frame "Task 2" {
                # "Robot responds when an obstacle (pick-up bin) is brought into\nthe sensor's field of view and the robot must make a pre-determined \nresponse such as reversing or any other action (team's choosing)."
                # ">>State Logic >>"
                n125 = Flush Queue(queue=w269) -> ()  [unwired: 1 in, 3 out]
                n126 = case shown="False" w268 {
                  tunnel: [w277 string[] ["Stop", "Hardware reset", "Software reset", "Motor control"]] -> w270
                  tunnel: w267 -> [w276 _]
                  frame False {
                    n127 = case shown="False" w276 {
                      tunnel: [string[] ["Stop", "Ultrasonic read", "Motor Control"] string[] ["Reverse", "Ultrasonic read", "Motor control"]] -> w277
                      frame False {
                      }
                      frame True {
                      }
                    }
                  }
                  frame True {
                  }
                }
                n128 = Select(t=TLB_MHL_States."Idle" ("Enum"), s=w268, f=TLB_MHL_States."Task 2" ("Enum")) -> (s? t:f=w273:T8)
                n129 = for {
                  shift-right: [w282] -> w272
                  shift-left: w271 -> [w283]
                  tunnel: w270 -> [w281] mode=indexing
                  n130 = Enqueue Element(queue=w283, element=w281) -> (queue out=w282:refnum<queue>)  [unwired: 2 in, 2 out]
                }
              }
              frame "Task 3" {
                # "Robot rotates at least 360 degrees within a 0.42m by a 0.3m space\n(footprint of robot's base must always be within the 0.42m x 0.3m\nboundary at all times during the rotation)."
                n131 = Greater Or Equal?(x=w284, y=360.0) -> (x >= y?=w288:bool)
                n132 = Flush Queue(queue=w287) -> ()  [unwired: 1 in, 3 out]
                n133 = Or(x=w288, y=w285) -> (x .or. y?=w289:bool)
                n134 = case shown="False" w289 {
                  tunnel: [string[] ["Rotate CW", "Motor Control"] string[] ["Software reset", "Hardware reset", "Motor Control"]] -> w295
                  frame False {
                  }
                  frame True {
                  }
                }
                n135 = for {
                  shift-right: [w297] -> w293
                  shift-left: w294 -> [w298]
                  tunnel: w295 -> [w296] mode=indexing
                  n136 = Enqueue Element(queue=w298, element=w296) -> (queue out=w297:refnum<queue>)  [unwired: 2 in, 2 out]
                }
                n137 = Select(t=TLB_MHL_States."Idle" ("Enum"), s=w289, f=TLB_MHL_States."Task 3" ("Enum")) -> (s? t:f=w290:T8)
              }
              frame "Task 4" {
                n138 = Flush Queue(queue=w304) -> ()  [unwired: 1 in, 3 out]
                n139 = Or(x=w302, y=w301) -> (x .or. y?=w303:bool)
                n140 = case shown="True" w303 {
                  tunnel: [string[] ["Forward", "Ultrasonic read", ""] string[] ["Stop", "Hardware reset", "Software reset", ""]] -> w305
                  frame False {
                  }
                  frame True {
                  }
                }
                n141 = for {
                  shift-right: [w316] -> w307
                  shift-left: w306 -> [w317]
                  tunnel: w305 -> [w315] mode=indexing
                  n142 = Enqueue Element(queue=w317, element=w315) -> (queue out=w316:refnum<queue>)  [unwired: 2 in, 2 out]
                }
                n143 = case shown="True" w301 {
                  tunnel: [TLB_MHL_States."Task 4a" ("Enum") TLB_MHL_States."Idle" ("Enum")] -> w309
                  frame False {
                  }
                  frame True {
                  }
                }
                n144 = Select(t=w309, s=w302, f=TLB_MHL_States."Task 4" ("Enum")) -> (s? t:f=w310:T8)
              }
              frame "Task 4a" {
                n145 = Greater Or Equal?(x=w318, y=0.5) -> (x >= y?=w321:bool)
                n146 = Flush Queue(queue=w319) -> ()  [unwired: 1 in, 3 out]
                n147 = case shown="True" w321 {
                  tunnel: [string[] ["Right", "Motor Control"] string[] ["Stop", "Hardware reset", "Software reset", "Motor Control"]] -> w324
                  frame False {
                  }
                  frame True {
                  }
                }
                n148 = for {
                  shift-right: [w331] -> w322
                  shift-left: w323 -> [w332]
                  tunnel: w324 -> [w330] mode=indexing
                  n149 = Enqueue Element(queue=w332, element=w330) -> (queue out=w331:refnum<queue>)  [unwired: 2 in, 2 out]
                }
                n150 = Select(t=TLB_MHL_States."Task 4b" ("Enum"), s=w321, f=TLB_MHL_States."Task 4a" ("Enum")) -> (s? t:f=w325:T8)
              }
              frame "Task 4b" {
                n151 = Flush Queue(queue=w334) -> ()  [unwired: 1 in, 3 out]
                n152 = Greater Or Equal?(x=w333, y=0.75) -> (x >= y?=w335:bool)
                n153 = case shown="False" w335 {
                  tunnel: [string[] ["Forward", "Motor control"] string[] ["Stop", "Hardware reset", "Software reset"]] -> w340
                  frame False {
                  }
                  frame True {
                  }
                }
                n154 = for {
                  shift-right: [w346] -> w338
                  shift-left: w339 -> [w347]
                  tunnel: w340 -> [w345] mode=indexing
                  n155 = Enqueue Element(queue=w347, element=w345) -> (queue out=w346:refnum<queue>)  [unwired: 2 in, 2 out]
                }
                n156 = Select(t=TLB_MHL_States."Task 4c" ("Enum"), s=w335, f=TLB_MHL_States."Task 4b" ("Enum")) -> (s? t:f=w337:T8)
              }
              frame "Task 4c" {
                n157 = Flush Queue(queue=w349) -> ()  [unwired: 1 in, 3 out]
                n158 = Less Or Equal?(x=w348, y=-0.65) -> (x <= y?=w350:bool)
                n159 = case shown="False" w350 {
                  tunnel: [string[] ["Left", "Motor Control"] string[] ["Stop", "Hardware reset", "Software reset", "Motor Control"]] -> w355
                  frame False {
                  }
                  frame True {
                  }
                }
                n160 = for {
                  shift-right: [w361] -> w352
                  shift-left: w353 -> [w362]
                  tunnel: w355 -> [w360] mode=indexing
                  n161 = Enqueue Element(queue=w362, element=w360) -> (queue out=w361:refnum<queue>)  [unwired: 2 in, 2 out]
                }
                n162 = Select(t=TLB_MHL_States."Task 4d" ("Enum"), s=w350, f=TLB_MHL_States."Task 4c" ("Enum")) -> (s? t:f=w354:T8)
              }
              frame "Task 4d" {
                n163 = Flush Queue(queue=w365) -> ()  [unwired: 1 in, 3 out]
                n164 = Or(x=w364, y=w363) -> (x .or. y?=w366:bool)
                n165 = case shown="True" w366 {
                  tunnel: [string[] ["Forward", "Ultrasonic Read", "Motor Control"] string[] ["Stop", "Hardware reset", "Software reset", "Motor Control"]] -> w370
                  frame False {
                  }
                  frame True {
                  }
                }
                n166 = for {
                  shift-right: [w376] -> w368
                  shift-left: w369 -> [w377]
                  tunnel: w370 -> [w375] mode=indexing
                  n167 = Enqueue Element(queue=w377, element=w375) -> (queue out=w376:refnum<queue>)  [unwired: 2 in, 2 out]
                }
                n168 = Select(t=TLB_MHL_States."Idle" ("Enum"), s=w366, f=TLB_MHL_States."Task 4d" ("Enum")) -> (s? t:f=w367:T8)
              }
              frame "Reset" {
                n169 = for {
                  shift-right: [w383] -> w378
                  shift-left: w379 -> [w384]
                  tunnel: string[] ["Software reset", "Hardware reset", "Motor Control"] -> [w382] mode=indexing
                  n170 = Enqueue Element(queue=w384, element=w382) -> (queue out=w383:refnum<queue>)  [unwired: 2 in, 2 out]
                }
              }
              frame "Wall follow mode" {
                n171 = Flush Queue(queue=w386) -> ()  [unwired: 1 in, 3 out]
                n172 = case shown="False" w385 {
                  tunnel: [string[] ["IR Sensor Read", "Calculate", "Forward", "Motor Control"] string[] ["Hardware reset", "Software reset", "Motor Control"]] -> w387
                  frame False {
                  }
                  frame True {
                  }
                }
                n173 = for {
                  shift-right: [w396] -> w389
                  shift-left: w388 -> [w397]
                  tunnel: w387 -> [w395] mode=indexing
                  n174 = Enqueue Element(queue=w397, element=w395) -> (queue out=w396:refnum<queue>)  [unwired: 2 in, 2 out]
                }
                n175 = Select(t=TLB_MHL_States."Idle" ("Enum"), s=w385, f=TLB_MHL_States."Wall follow mode" ("Enum")) -> (s? t:f=w391:T8)
              }
              frame "Autodrive" {
                # ">>>Return to idle event>>>"
                n176 = Flush Queue(queue=w405) -> ()  [unwired: 1 in, 3 out]
                n177 = Boolean To (0,1)(Boolean=w399) -> (0, 1=w404:i16)
                n178 = Boolean To (0,1)(Boolean=w398) -> (0, 1=w403:i16)
                n179 = formula code="int8  out;\nif (detect == 0 && stop == 0)\nout = 0;\n\nelse if (detect == 1 && stop == 0)\nout = 1;\n\nelse if (detect == 0 && stop == 1)\nout = 2;\n\nelse\nout = 0;"("stop"=w404, "detect"=w403) -> ("out"=w400:i8)
                n180 = case shown="0, Default" w400 {
                  tunnel: [string[] ["Forward", "Ultrasonic read"] string[] ["Hardware reset", "Software reset", "Rotate Clockwise", ""] string[] ["Stop", "", "Software reset", "Motor Control"]] -> w402
                  frame 0, Default {
                  }
                  frame 1 {
                  }
                  frame 2 {
                  }
                }
                n181 = for {
                  shift-right: [w415] -> w407
                  shift-left: w406 -> [w416]
                  tunnel: w402 -> [w414] mode=indexing
                  n182 = Enqueue Element(queue=w416, element=w414) -> (queue out=w415:refnum<queue>)  [unwired: 2 in, 2 out]
                }
                n183 = case shown="0, Default" w400 {
                  tunnel: [TLB_MHL_States."Autodrive" ("Enum") TLB_MHL_States."Autodrive a" ("Enum") TLB_MHL_States."Idle" ("Enum")] -> w401
                  frame 0, Default {
                  }
                  frame 1 {
                  }
                  frame 2 {
                  }
                }
              }
              frame "Autodrive a" {
                n184 = Greater Or Equal?(x=w417, y=80.0) -> (x >= y?=w419:bool)
                n185 = Or(x=w418, y=w419) -> (x .or. y?=w420:bool)
                n186 = case shown="True" w420 {
                  tunnel: [string[] ["Rotate CW", "Ultrasonic read", ""] string[] ["Stop", "", "Software reset", ""]] -> w428
                  frame False {
                  }
                  frame True {
                  }
                }
                n187 = for {
                  shift-right: [w434] -> w430
                  shift-left: w429 -> [w435]
                  tunnel: w428 -> [w433] mode=indexing
                  n188 = Enqueue Element(queue=w435, element=w433) -> (queue out=w434:refnum<queue>)  [unwired: 2 in, 2 out]
                }
                n189 = Or(x=w418, y=w419) -> (x .or. y?=w421:bool)
                n190 = Select(t=TLB_MHL_States."Idle" ("Enum"), s=w418, f=TLB_MHL_States."Autodrive" ("Enum")) -> (s? t:f=w424:T8)
                n191 = Select(t=w424, s=w421, f=TLB_MHL_States."Autodrive a" ("Enum")) -> (s? t:f=w426:T8)
              }
              frame "Acquire image" {
                n192 = Flush Queue(queue=w437) -> ()  [unwired: 1 in, 3 out]
                n193 = case shown="False" w436 {
                  tunnel: [string[] ["Cam Acq"] string[] ["Hardware reset", "Software reset", "Cam Exit", ""]] -> w441
                  frame False {
                  }
                  frame True {
                  }
                }
                n194 = for {
                  shift-right: [w447] -> w439
                  shift-left: w440 -> [w448]
                  tunnel: w441 -> [w446] mode=indexing
                  n195 = Enqueue Element(queue=w448, element=w446) -> (queue out=w447:refnum<queue>)  [unwired: 2 in, 2 out]
                }
                n196 = Select(t=TLB_MHL_States."Idle" ("Enum"), s=w436, f=TLB_MHL_States."Acquire image" ("Enum")) -> (s? t:f=w438:T8)
              }
              frame "Processing" {
              }
              frame "Shutdown" {
                # ">>State Logic >>"
                n197 = for {
                  shift-right: [w456] -> w451
                  shift-left: w452 -> [w457]
                  tunnel: string[] ["Software reset", "Hardware reset", "Motor Control", "Cam Exit", "Pre-Exit", "Exit"] -> [w455] mode=indexing
                  n198 = Enqueue Element(queue=w457, element=w455) -> (queue out=w456:refnum<queue>)  [unwired: 2 in, 2 out]
                }
              }
              frame "None" {
              }
            }
          }
        }
        "Decision" <- w129
      }
      n199 = call <vilib>:"DIO Close.vi"("error in (no error)"=w10, "DIO Info In"=w12) -> ()  [unwired: 9 in, 1 out]
      n200 = call <vilib>:"DIO Close.vi"("error in (no error)"=w6, "DIO Info In"=w9) -> ()  [unwired: 9 in, 1 out]
      n201 = Merge Errors "Merge Errors"(w39, w38) -> (w20:errorcluster)
      n202 = Merge Errors(w24, w20) -> (w15:errorcluster)
      n203 = Destroy User Event(user event=w42, error in=w15) -> ()  [unwired: 1 out]
      n204 = Destroy User Event(user event=w43, error in=w15) -> ()  [unwired: 1 out]
      n205 = Unregister For Events(event registration refnum=w34, error in=w15) -> ()  [unwired: 1 out]
      n206 = Release Queue(queue=w17, error in (no error)=w15) -> (error out=→"error out":errorcluster)  [unwired: 1 in, 2 out]
      n207 = call <vilib>:"NavX Close.vi"("NavX Info In"=w14) -> ()  [unwired: 10 in, 1 out]
      n208 = Release Queue(queue=w33, error in (no error)=w15) -> ()  [unwired: 1 in, 3 out]
    }
    frame #2 {
      n209 = Wait (ms)(milliseconds to wait=u32 100) -> ()  [unwired: 1 out]
      n210 = call "PID Movement final version.vi"("Direction"=T3."Init") -> ()  [unwired: 3 in, 2 out]
    }
    frame #3 {
    }
  }
